vi "Read Requirements.vi"(8 "error in (no error)":errorcluster, 11 "Requirements file":path) -> (0 "error out":errorcluster, 2 "# Requirements":i32, 3 "Requirements":string[](array[string]))   [LabVIEW 2018, in "Covers-o-meter.lvlib"]
uses:
  Covers-o-meter.lvlib
  <vilib>/Utility/error.llb/whitespace.ctl
  <vilib>/Utility/file.llb/Read Delimited Spreadsheet (string).vi
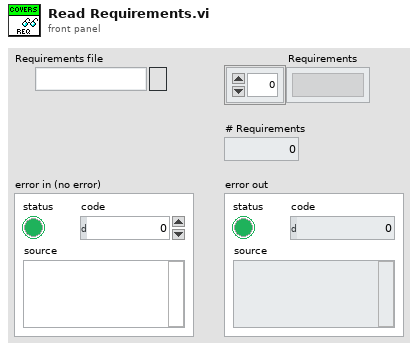
[diagram p1: front panel]
types:
  T1 = typedef "whitespace.ctl" = u16
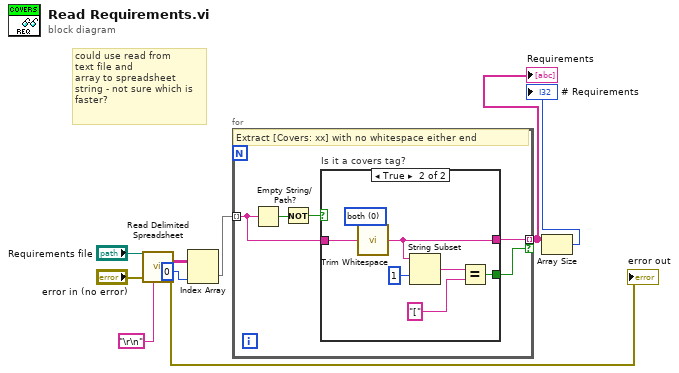
[diagram p0: block diagram]
diagram:
  # "could use read from\ntext file and \narray to spreadsheet\nstring - not sure which is\nfaster?"
  n1 = call-poly <vilib>:"Read Delimited Spreadsheet.vi"("file path (dialog if empty)"="Requirements file", "error in (no error)"="error in (no error)", "delimiter (\\t)"="\r\n") -> ("all rows"=w2:string[][], "error out"=→"error out":errorcluster)  [unwired: 7 in, 4 out]
  n2 = Index Array(array=w2, index (col)=0 ("disabled index (col)")) -> (element=w1:string[])  [unwired: 1 in]
  n3 = for {
    tunnel: w1 -> [w11] mode=indexing
    tunnel: [w12] -> w8 mode=indexing if=w10
    # "Extract [Covers: xx] with no whitespace either end"
    n4 = Empty String/Path?(string/path=w11) -> (empty?=w14:bool)
    n5 = Not(x=w14) -> (.not. x?=w13:bool)
    n6 = case "Is it a covers tag?" shown="True" w13 {
      tunnel: w11 -> [w15 w22]
      tunnel: [w15 w16] -> w12
      tunnel: [_ w18] -> w10
      frame False {
      }
      frame True {
        w21 = T1 0 items=["both", "start of string", "end of string"] ("location (both)")
        n7 = call <vilib>:"Trim Whitespace.vi"("string"=w22, "location (both)"=w21) -> ("trimmed string"=w16:string)
        n8 = String Subset(string=w16, length (rest)=1 ("length (rest)")) -> (substring=w19:string)  [unwired: 1 in]
        n9 = Equal?(x=w19, y="[" ("x")) -> (x = y?=w18:bool)
      }
    }
  }
  "Requirements" <- w8
  n10 = Array Size(array=w8) -> (size(s)=→"# Requirements":i32)
